vi "Scale Params.vi"(7 "SensorList (Auto)":refnum<class "SensorList.lvclass">, 8 "error in (no error)":errorcluster, 11 "Scale in":refnum<class "Scale.lvclass">) -> (0 "error out":errorcluster, 1 "Scale Params":dbl[](array[numeric]), 2 "Scale Type":T1, 3 "Scale out":refnum<class "Scale.lvclass">)   [LabVIEW 2020, in "VolatusConfig.lvlib" / "Scale.lvclass"]
uses:
  Scale.lvclass
  C:/dev/lv20CE/relink/lv-volatus/VolatusConfig/VolatusConfigElement/VolatusConfigElement.lvclass
  SensorList/SensorList.lvclass
  Scale Type.ctl
  VolatusConfigElement/VolatusConfigElement.lvclass/VolatusConfigElement.ctl
  VolatusConfigElement/Element.vi
  Scale.lvclass/Scale.ctl
  VolatusConfigElement/VolatusConfigElement.lvclass
  lv-cdm/CDM-Config/Config Element/Config Element.lvclass
  VolatusConfig.lvlib
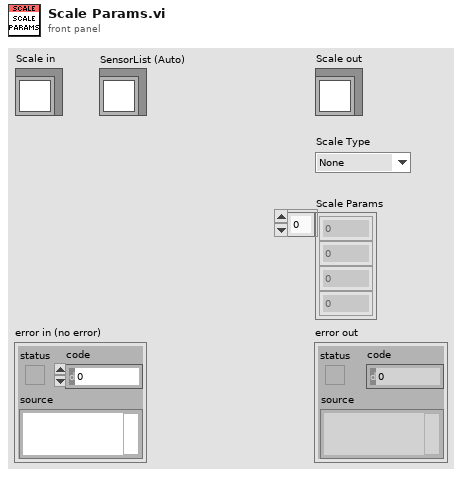
[diagram p1: front panel]
types:
  T1 = typedef "VolatusConfig.lvlib/Scale Type.ctl" = enum16{"None", "Sensor", "Polynomial", "Threshold", "Invert Bool"}
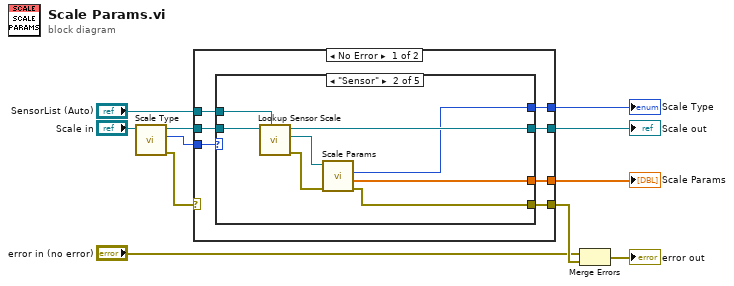
[diagram p0: block diagram]
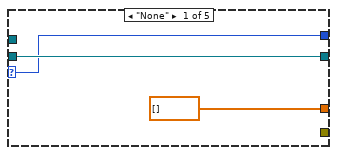
[diagram p2: hidden frame]
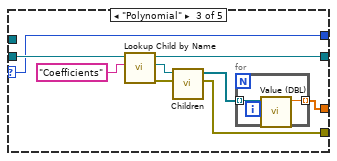
[diagram p3: hidden frame]
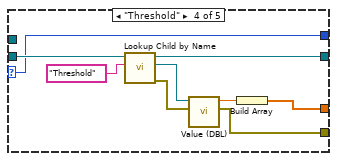
[diagram p4: hidden frame]
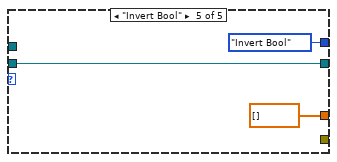
[diagram p5: hidden frame]
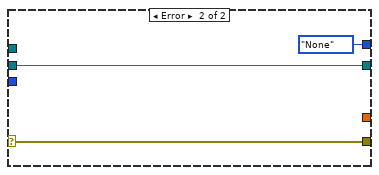
[diagram p6: hidden frame]
diagram:
  n1 = call "Scale Type.vi"("Scale in"="Scale in") -> ("error out"=w11:errorcluster, "Scale Type"=w2:T1, "Scale out"=w9:refnum<class "Scale.lvclass">)  [unwired: 8 in]
  n2 = case shown="No Error" w11 {
    selector: w11 -> [_ w55]
    tunnel: [w18 w55] -> w10
    tunnel: w9 -> [w17 w54]
    tunnel: [w16 w54] -> w7
    tunnel: [w15 _] -> w4
    tunnel: w2 -> [w14 _]
    tunnel: "SensorList (Auto)" -> [w13 _]
    tunnel: [w12 Scale_Type."None" ("Scale Type")] -> w1
    frame No Error {
      n3 = case shown="\"Sensor\"" w14 {
        selector: w14 -> [w19 _ w30 w41 _]
        tunnel: [_ w25 w33 w43 _] -> w18
        tunnel: w17 -> [w21 w29 w38 w49 w51]
        tunnel: [w21 w28 w32 w47 w51] -> w16
        tunnel: [dbl[] [] w23 w31 w42 dbl[] [] ("Scale Params")] -> w15
        tunnel: w13 -> [_ w24 _ _ _]
        tunnel: [w19 w22 w30 w41 Scale_Type."Invert Bool" ("Scale Type")] -> w12
        frame "None" {
        }
        frame "Sensor" {
          n4 = call "Lookup Sensor Scale.vi"("SensorList"=w24, "Scale in"=w29) -> ("error out"=w26:errorcluster, "Sensor Scale"=w27:refnum<class "Scale.lvclass">, "Scale out"=w28:refnum<class "Scale.lvclass">)  [unwired: 7 in]
          n5 = call "Scale Params.vi"("error in (no error)"=w26, "Scale in"=w27) -> ("error out"=w25:errorcluster, "Scale Params"=w23:dbl[], "Scale Type"=w22:T1)  [unwired: 6 in, 1 out]
        }
        frame "Polynomial" {
          n6 = call "Lookup Child by Name.vi"("Child Name"="Coefficients", "VolatusConfigElement in"=w38) -> ("error out"=w36:errorcluster, "Child"=w35:refnum<class "Config Element.lvclass">, "VolatusConfigElement out"=w32:refnum<class "Scale.lvclass">)  [unwired: 6 in, 1 out]
          n7 = call "Children.vi"("error in (no error)"=w36, "Config Element in"=w35) -> ("error out"=w33:errorcluster, "Elements"=w34:refnum<class "Config Element.lvclass">[])  [unwired: 8 in]
          n8 = for {
            tunnel: w34 -> [w40] mode=indexing
            tunnel: [w39] -> w31 mode=indexing
            n9 = call "Value (DBL).vi"("Config Element in"=w40) -> ("DBL Value"=w39:dbl)  [unwired: 9 in, 1 out]
          }
        }
        frame "Threshold" {
          n10 = call "Lookup Child by Name.vi"("Child Name"="Threshold", "VolatusConfigElement in"=w49) -> ("error out"=w44:errorcluster, "Child"=w45:refnum<class "Config Element.lvclass">, "VolatusConfigElement out"=w47:refnum<class "Scale.lvclass">)  [unwired: 6 in, 1 out]
          n11 = call "Value (DBL).vi"("error in (no error)"=w44, "Config Element in"=w45) -> ("error out"=w43:errorcluster, "DBL Value"=w46:dbl)  [unwired: 8 in]
          n12 = Build Array(w46) -> (w42:dbl[])
        }
        frame "Invert Bool" {
        }
      }
    }
    frame Error {
    }
  }
  "Scale out" <- w7
  "Scale Params" <- w4
  "Scale Type" <- w1
  n13 = Merge Errors("error in (no error)", w10) -> (→"error out":errorcluster)
